vi "global mass.vi"() -> ()   [LabVIEW 2018]
panel:
  in  "1/B ave. mass":dbl[](array[numeric]) format="%.2f"
  in  "mass":dbl[][](array[numeric]) format="%.2f"
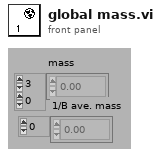
[diagram p1: front panel]
diagram:
